vi "Shutdown.vi"(8 "error in (no error)":errorcluster, 11 "Thermal Camera in":refnum<class "Thermal Camera.lvclass">) -> (0 "error out":errorcluster, 3 "Thermal Camera out":refnum<class "Thermal Camera.lvclass">)   [LabVIEW 2018, in "Thermal Camera.lvlib" / "Thermal Camera.lvclass"]
uses:
  Thermal Camera.lvclass
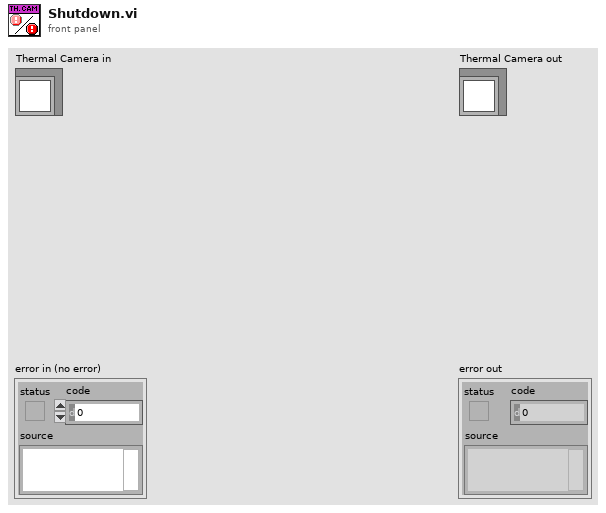
[diagram p1: front panel]
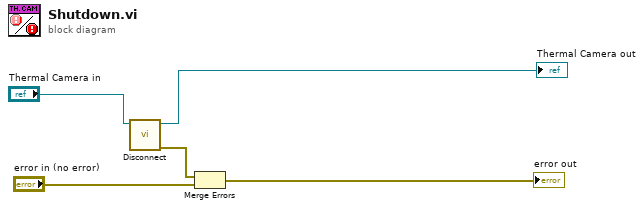
[diagram p0: block diagram]
diagram:
  n1 = call-dynamic "Disconnect.vi"("Thermal Camera in"="Thermal Camera in") -> ("error out"=w4:errorcluster, "Thermal Camera out"=→"Thermal Camera out":refnum<class "Thermal Camera.lvclass">)  [unwired: 9 in]
  n2 = Merge Errors(w4, "error in (no error)") -> (→"error out":errorcluster)
